vi "LR-700.vi"() -> ()   [LabVIEW 2020]
panel:
  out "cluster":T1 {"X Set" format="%.5e"; "R Set" format="%.5e"; "ÆX" format="%.5e"; "ÆR" format="%.5e"; "X" format="%.5e"; "R" format="%.5e"}
  in  "Open Loop Heat":dbl(knob) min=0.0 max=99.9 step=0.1 scale=0.0..99.9 scale format="%.1f"
  in  "Loop Control":u8(slide) max=2 step=1 scale=0.0..2.0
  in  "Heater Option":bool
  in  "Heater Gain":T2(ring)
  out "Overloads":T3
  in  "heater Hold":bool
  in  "Heater Input Filter":T4(ring)
  in  "Offset Value":dbl(knob) min=-1.99999 max=1.99999 step=1e-05 scale=-2.0..2.0 scale format="%.1f"
  in  "Offset":T5(ring)
  in  "Mode":enum16{"X1", "X10"}(ring)
  in  "GPIB Address":refnum<visa-resource-name>
  in  "% of Full Excitation":u16(knob)=100 min=5 max=100 step=1 scale=0.0..100.0
  in  "Range":T6(ring)=enum."2 k½"
  in  "Top":T7(ring)
  in  "Bottom":T7(ring)=enum."X Measurement"
  in  "Sensor #":u32=1 min=1 max=99 step=1
  in  "Heater Display":T8(ring)=enum."Bar Graph % Current"
  out "?":string[](array[string])
  in  "Heater Control":enum16{"D", "DI", "I", "P", "PD", "PI", "PID"}(ring)=enum."PD"
  in  "heater":bool
  in  "Full Excitation":T9(ring)=enum."2 mV"
  in  "Filter":T10(ring)=enum."1.6 Seconds"
  # "Display"
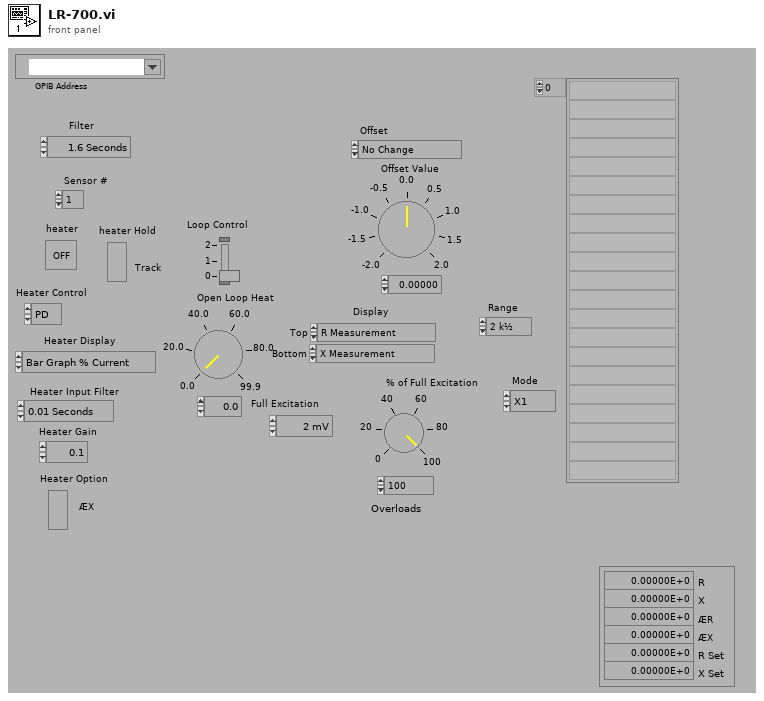
[diagram p1: front panel]
types:
  T1 = cluster{"R":dbl, "X":dbl, "ÆR":dbl, "ÆX":dbl, "R Set":dbl, "X Set":dbl}
  T2 = enum16{"0.1", "0.2", "0.5", "1", "2", "5", "10", "20", "50", "100", "200", "500", "1000", "2000", "5000"}
  T3 = cluster{bool, bool, bool, bool, bool, bool, bool, bool}
  T4 = enum16{"0.01 Seconds", "0.1 Seconds", "0.3 Seconds", "1 Second", "3 Seconds", "10 Seconds", "30 Seconds"}
  T5 = enum16{"No Change", "Zero Offset", "Offset Current Value", "Set R Offest to Value", "Set X Offset to Value"}
  T6 = enum16{"2 m½", "20 m½", "200 m½", "2 ½", "20 ½", "200 ½", "2 k½", "20 k½", "200 k½", "2 M½"}
  T7 = enum16{"R Measurement", "X Measurement", "ÆR/10ÆR Measurement", "ÆX/10ÆX Measurement", "R Setting Value", "X Setting Value", "% Excitation Setting", "Filter Setting", "Temperature Controller", "Special Function"}
  T8 = enum16{"Numeric Voltage", "Bar Graph Voltage", "Numeric % Current", "Bar Graph % Current"}
  T9 = enum16{"20 µV", "60 µV", "200 µV", "600 µV", "2 mV", "6 mV", "20 mV"}
  T10 = enum16{"0.2 Seconds", "0.4 Seconds", "0.6 Seconds", "1 Second", "1.6 Seconds", "2 Seconds", "3 Seconds", "5 Seconds", "7 Seconds", "10 Seconds", "15 Seconds", "20 Seconds", "30 Seconds", "45 Seconds", "1 Minute", "1.5 Minutes", "2 Minutes", "3 Minutes", "5 Minutes", "7 Minutes", "10 Minutes", "15 Minutes", "20 Minutes", "30 Minutes"}
  T11 = cluster{"Boolean array[0]":bool, "Boolean array[1]":bool, "Boolean array[2]":bool, "Boolean array[3]":bool, "Boolean array[4]":bool, "Boolean array[5]":bool, "Boolean array[6]":bool, "Boolean array[7]":bool}
  T12 = cluster{"[0]":u16, "[1]":u16, "[2]":u16, "[3]":u16, "[4]":u16, "[5]":u16, "[6]":u16, "[7]":u16, "[8]":u16}
  T13 = cluster{"[0]":dbl, "[1]":dbl, "[2]":dbl, "[3]":dbl, "[4]":dbl, "[5]":dbl}
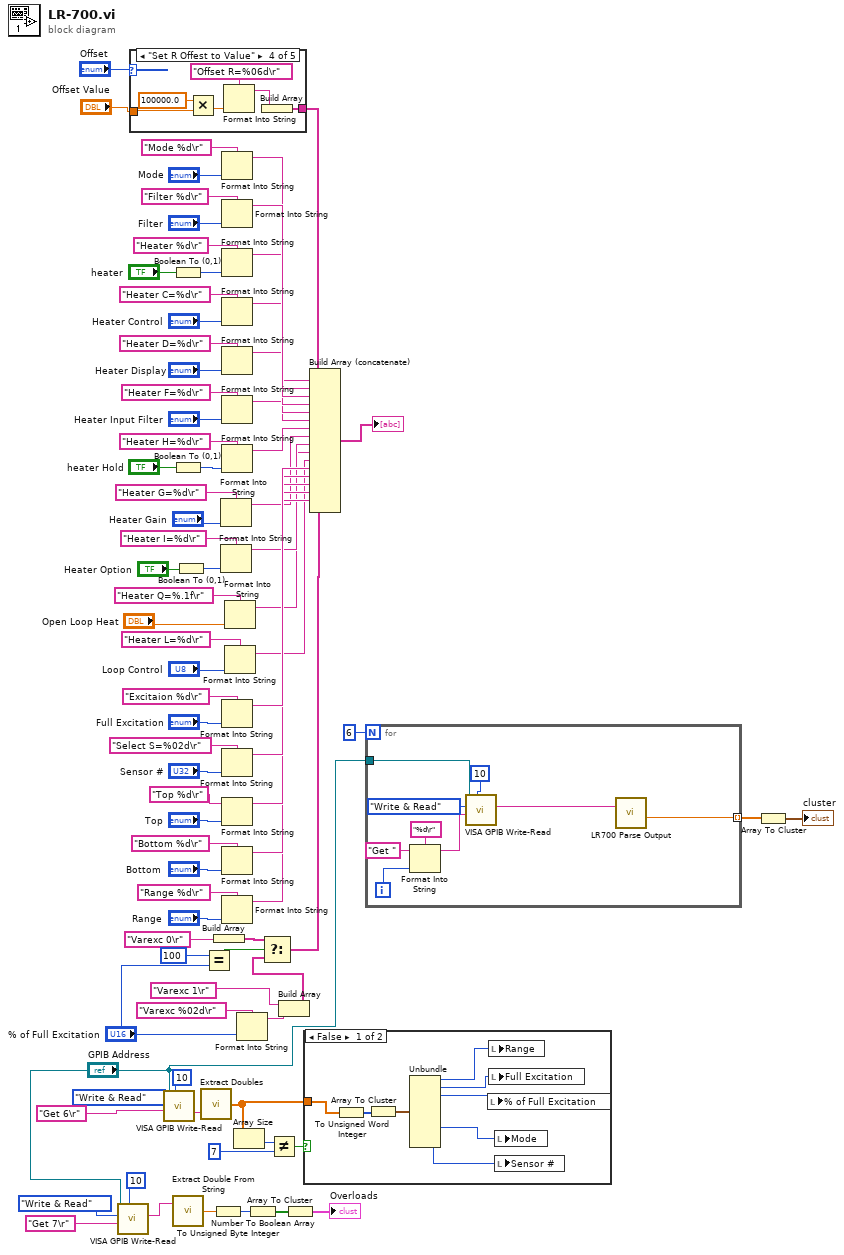
[diagram p0: block diagram]
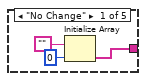
[diagram p3: hidden frame]
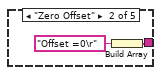
[diagram p4: hidden frame]
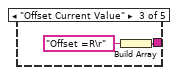
[diagram p5: hidden frame]
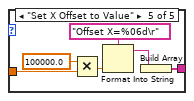
[diagram p6: hidden frame]
diagram:
  n1 = call "VISA GPIB Write-Read.vi"("Wait (ms)"=u32 10 ("wait (mS)"), "Command"="Get 7\r", "Action"=enum16{"Write", "Read", "Write & Read"}."Write & Read", "VISA resource name"="GPIB Address") -> ("String Returned"=w26:string)  [unwired: 4 in, 3 out]
  n2 = case shown="\"Set R Offest to Value\"" "Offset" {
    tunnel: [w86 w89 w91 w98 w104] -> w42
    tunnel: "Offset Value" -> [_ _ _ w93 w100]
    frame "No Change" {
      n3 = Initialize Array("", 0) -> (w86:string[])
    }
    frame "Zero Offset" {
      n4 = Build Array("Offset =0\r") -> (w89:string[])
    }
    frame "Offset Current Value" {
      n5 = Build Array("Offset =R\r") -> (w91:string[])
    }
    frame "Set R Offest to Value" {
      n6 = Multiply(x=100000.0, y=w93) -> (x*y=w94:dbl)
      n7 = Format Into String(format string="Offset R=%06d\r", w94) -> (resulting string=w97:string)  [unwired: 2 in, 1 out]
      n8 = Build Array(w97) -> (w98:string[])
    }
    frame "Set X Offset to Value" {
      n9 = Multiply(x=100000.0, y=w100) -> (x*y=w101:dbl)
      n10 = Format Into String(format string="Offset X=%06d\r", w101) -> (resulting string=w103:string)  [unwired: 2 in, 1 out]
      n11 = Build Array(w103) -> (w104:string[])
    }
  }
  n12 = call "VISA GPIB Write-Read.vi"("Wait (ms)"=u32 10 ("wait (mS)"), "Command"="Get 6\r", "Action"=enum16{"Write", "Read", "Write & Read"}."Write & Read", "VISA resource name"="GPIB Address") -> ("String Returned"=w47:string)  [unwired: 4 in, 3 out]
  n13 = Boolean To (0,1)(Boolean="heater") -> (0, 1=w81:i16)
  n14 = Boolean To (0,1)(Boolean="heater Hold") -> (0, 1=w32:i16)
  n15 = call "Extract Double From String.vi"("string"=w26) -> ("floating pt. number"=w24:dbl)  [unwired: 1 in, 2 out]
  n16 = Boolean To (0,1)(Boolean="Heater Option") -> (0, 1=w17:i16)
  n17 = call "Extract Doubles.vi"("String"=w47) -> ("Data"=w30:dbl[])  [unwired: 1 in]
  n18 = Equal?(x=u16 100, y="% of Full Excitation") -> (x = y?=w56:bool)
  n19 = To Unsigned Byte Integer(number=w24) -> (unsigned 8bit integer=w23:u8)
  n20 = Build Array("Varexc 0\r") -> (w57:string[])
  n21 = Format Into String(format string="Heater G=%d\r", "Heater Gain") -> (resulting string=w13:string)  [unwired: 2 in, 1 out]
  n22 = Format Into String(format string="Heater I=%d\r", w17) -> (resulting string=w12:string)  [unwired: 2 in, 1 out]
  n23 = Format Into String(format string="Mode %d\r", "Mode") -> (resulting string=w44:string)  [unwired: 2 in, 1 out]
  n24 = Format Into String(format string="Filter %d\r", "Filter") -> (resulting string=w76:string)  [unwired: 2 in, 1 out]
  n25 = Format Into String(format string="Heater %d\r", w81) -> (resulting string=w75:string)  [unwired: 2 in, 1 out]
  n26 = Format Into String(format string="Heater C=%d\r", "Heater Control") -> (resulting string=w74:string)  [unwired: 2 in, 1 out]
  n27 = Format Into String(format string="Heater D=%d\r", "Heater Display") -> (resulting string=w36:string)  [unwired: 2 in, 1 out]
  n28 = Format Into String(format string="Heater F=%d\r", "Heater Input Filter") -> (resulting string=w35:string)  [unwired: 2 in, 1 out]
  n29 = Format Into String(format string="Heater H=%d\r", w32) -> (resulting string=w31:string)  [unwired: 2 in, 1 out]
  n30 = Format Into String(format string="Excitaion %d\r", "Full Excitation") -> (resulting string=w73:string)  [unwired: 2 in, 1 out]
  n31 = Format Into String(format string="Select S=%02d\r", "Sensor #") -> (resulting string=w69:string)  [unwired: 2 in, 1 out]
  n32 = Format Into String(format string="Top %d\r", "Top") -> (resulting string=w64:string)  [unwired: 2 in, 1 out]
  n33 = Format Into String(format string="Bottom %d\r", "Bottom") -> (resulting string=w63:string)  [unwired: 2 in, 1 out]
  n34 = Format Into String(format string="Range %d\r", "Range") -> (resulting string=w60:string)  [unwired: 2 in, 1 out]
  n35 = Format Into String(format string="Heater Q=%.1f\r", "Open Loop Heat") -> (resulting string=w8:string)  [unwired: 2 in, 1 out]
  n36 = Format Into String(format string="Heater L=%d\r", "Loop Control") -> (resulting string=w11:string)  [unwired: 2 in, 1 out]
  n37 = Array Size(array=w30) -> (size(s)=w29:i32)
  n38 = Format Into String(format string="Varexc %02d\r", "% of Full Excitation") -> (resulting string=w53:string)  [unwired: 2 in, 1 out]
  n39 = Number To Boolean Array(number=w23) -> (Boolean array=w22:bool[])
  n40 = Not Equal?(x=w29, y=7) -> (x != y?=w27:bool)
  n41 = Build Array("Varexc 1\r", w53) -> (w51:string[])
  n42 = Select(t=w57, s=w56, f=w51) -> (s? t:f=w50:string[])
  n43 = Array To Cluster(array=w22) -> (cluster=→"Overloads":T11)
  n44 = case shown="False" w27 {
    tunnel: w30 -> [w112 _]
    frame False {
      n45 = To Unsigned Word Integer(number=w112) -> (unsigned 16bit integer=w107:u16[])
      n46 = Array To Cluster(array=w107) -> (cluster=w108:T12)
      n47 = Unbundle(w108) -> ("[0]"=w109:u16, "[1]"=w110:u16, "[2]"=w111:u16, "[6]"=w105:u16, "[8]"=w106:u16)  [unwired: 4 out]
      n48 = local write "% of Full Excitation"(w111) -> ()
      n49 = local write "Range"(w109) -> ()
      n50 = local write "Full Excitation"(w110) -> ()
      n51 = local write "Mode"(w105) -> ()
      n52 = local write "Sensor #"(w106) -> ()
    }
    frame True {
    }
  }
  n53 = Build Array (concatenate)(w42, w44, w76, w75, w74, w36, w35, w31, w13, w12, w8, w11, w73, w69, w64, w63, w60, w50) -> (→"?":string[])
  n54 = for {
    N: 6 -> [_]
    tunnel: "GPIB Address" -> [w121]
    tunnel: [w120] -> w6 mode=indexing
    i -> [w115]
    n55 = Format Into String(format string="%d\r", initial string="Get ", w115) -> (resulting string=w117:string)  [unwired: 1 in, 1 out]
    n56 = call "VISA GPIB Write-Read.vi"("Wait (ms)"=u32 10 ("wait (mS)"), "Command"=w117, "Action"=enum16{"Write", "Read", "Write & Read"}."Write & Read", "VISA resource name"=w121) -> ("String Returned"=w119:string)  [unwired: 4 in, 3 out]
    n57 = call "LR700 Parse Output.vi"("String Read"=w119) -> (0:w120:dbl)
  }
  n58 = Array To Cluster(array=w6) -> (cluster=→"cluster":T13)
